vi "W2Q1.vi"() -> ()   [LabVIEW 2023]
panel:
  out "Numeric":i32
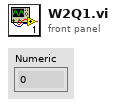
[diagram p1: front panel]
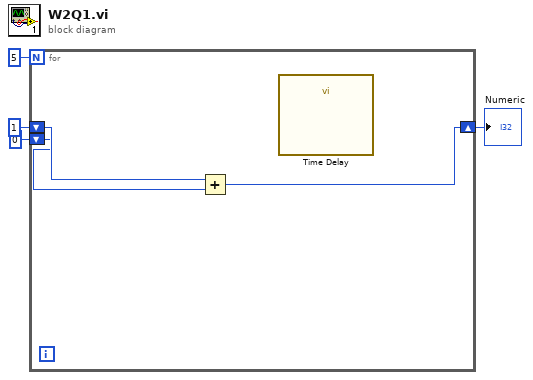
[diagram p0: block diagram]
diagram:
  n1 = for {
    N: 5 -> [_]
    shift-right: [w6] -> w2
    shift-left: 1 -> [w7]
    shift-left: 0 -> [w5]
    n2 = Add(x=w7, y=w5) -> (x+y=w6:i32)
    n3 = call "Time Delay"() -> ()  [unwired: 11 in, 1 out]
  }
  "Numeric" <- w2
